vi "LV to ITX  Retrieve Equation.vi"(0 "File or Folder Path":path=path "\\\\TILES\\Data/SA02777G.graphene.20150414/12 - sweep B +-2T, step Vsg", 5 "offset":i32, 7 "length":i32=10, 9 "index":T1={"a"=3, "b"=5, "c"=7, "d"=9, "f"=2, "N1"=2, "N2"=0, "N3"=0, "N4"=0}) -> (4 "y1 vs f":cluster{dbl[], dbl[]}[](graph), 6 "y2 vs f":cluster{dbl[], dbl[]}[](graph), 8 "2D":dbl[][](graph), 10 "N":cluster{"N1":dbl, "N2":dbl, "N3":dbl, "N4":dbl}={"N1"=0.0, "N2"=3512286493.887331, "N3"=3512286493.887331, "N4"=3512286493.887331} {"N4" format="%#_6p"; "N3" format="%#_6p"; "N2" format="%#_6p"; "N1" format="%#_6p"}, 14 "Comments":string="sweep Vsg (22): 750mV to -500mV 50mV steps\r\n\r\n\r\n\r\n\r\n\r\n\r\n\r\n\r\n\r\n\r\n\r\n\r\n\r\n\r\nB=0T to 2T to -2T to 0T, 0.0104 A/s\r\n\r\n\r\n\r\n\r\n\r\n\r\n\r\n\r\n\r\n\r\n\r\n\r\n\r\n\r\n\r\n\r\n\r\n\r\n\r\n\r\n\r\n\r\n\r\n\r\n\r\n\r\n\r\n\r\n\r\nlockin\r\n\r\n\r\n\r\n\r\n\r\n\r\n\r\n\r\n\r\n\r\n\r\n\r\n\r\n\r\n0: 1\r\n\r\n\r\n\r\n\r\n\r\n\r\n\r\n\r\n\r\n\r\n\r\n\r\n\r\n\r\n1: 3\r\n\r\n\r\n\r\n\r\n\r\n\r\n\r\n\r\n\r\n\r\n\r\n\r\n\r\n\r\n2: 4, current\r\n\r\n\r\n\r\n\r\n\r\n\r\n\r\n\r\n\r\n\r\n\r\n\r\n\r\n\r\n3: 5\r\n\r\n\r\n\r\n\r\n\r\n\r\n\r\n\r\n\r\n\r\n\r\n\r\n\r\n\r\n4: 27\r\n\r\n\r\n\r\n\r\n\r\n\r\n\r\n\r\n\r\n\r\n\r\n\r\n\r\n\r\n5: 28, current, 8mV AC\r\n\r\n\r\n\r\n\r\n\r\n\r\n\r\n\r\n\r\n\r\n\r\n\r\n\r\n\r\nappliedVsg= 0.300000\r\n\r\n\r\n\r\n\r\n\r\n\r\n\r\n\r\n\r\n\r\n\r\n\r\n\r\n\r\n")   [LabVIEW 2013]
uses:
  <vilib>/Utility/miscctls.llb/LVOffsetAndMultiplierTypeDef.ctl
  <vilib>/gmath/NI_Gmath.lvlib
panel:
  in  "2D graph:\non = y1, off = y2":bool=TRUE
  in  "reverse arrays?":bool[](array[boolean])
  in  "header length":i32=11
  in  "Normalize MR?":bool=TRUE
  in  "threshold y":dbl
  in  "data length":i32=2500
  in  "data index":i32=1400
  in  "string formula = ON\nblock diagram formula = OFF":bool
  in  "Enum":enum16{"ITX", "ITX w/ 2D", "DAT"}(ring)=enum."DAT"
  in  "formula":string="y1 = (a-b)/c;\ny2 = (b-d)/c;"
  in  "D  is time?":bool
  in  "B is time?":bool
  out "time":string[][](table)=[["4/18/2015", "12:40 PM"], ["4/18/2015", "5:05 PM"], ["4/18/2015", "10:04 PM"], ["4/18/2015", "11:37 PM"], ["4/19/2015", "1:07 AM"], ["4/19/2015", "2:37 AM"], ["4/19/2015", "4:07 AM"], ["4/19/2015", "5:37 AM"], ["4/19/2015", "7:08 AM"], ["4/19/2015", "8:38 AM"]]
  in  "Use Folder Index File?":bool
  in  "Generate Folder Index File?":bool
  in  "Ez name":string="Ez name"
  in  "Ey name":string="Ey name"
  in  "Ex name":string="Ex name"
  in  "C y name":string="C y name"
  in  "D x name":string="D x name"
  in  "A y name":string="A y name"
  in  "B x name":string="B x name"
  out "Index, Wavenames":string[][](table)=[["0", "time"], ["1", "temp"], ["2", "Bfield"], ["3", "X0"], ["4", "Y0"], ["5", "X1"], ["6", "Y1"], ["7", "X2"], ["8", "Y2"], ["9", "X3"], ["10", "Y3"], ["11", "X4"], ["12", "Y4"], ["13", "X5"], ["", "Y5"]]
  in  "recolor traces?":bool=TRUE
  in  "Ex":T2={"Offset"=0.0, "Multiplier"=1.0}
  in  "Ey":T2={"Offset"=0.0, "Multiplier"=1.0}
  out "Path":path=path "\\\\TILES\\Data/SA02777G.graphene.20150414/12 - sweep B +-2T, step Vsg/SA02777G.graphene.20150414.000009.dat"
  out "counter":i32=9
  in  "pattern":string="*.dat"
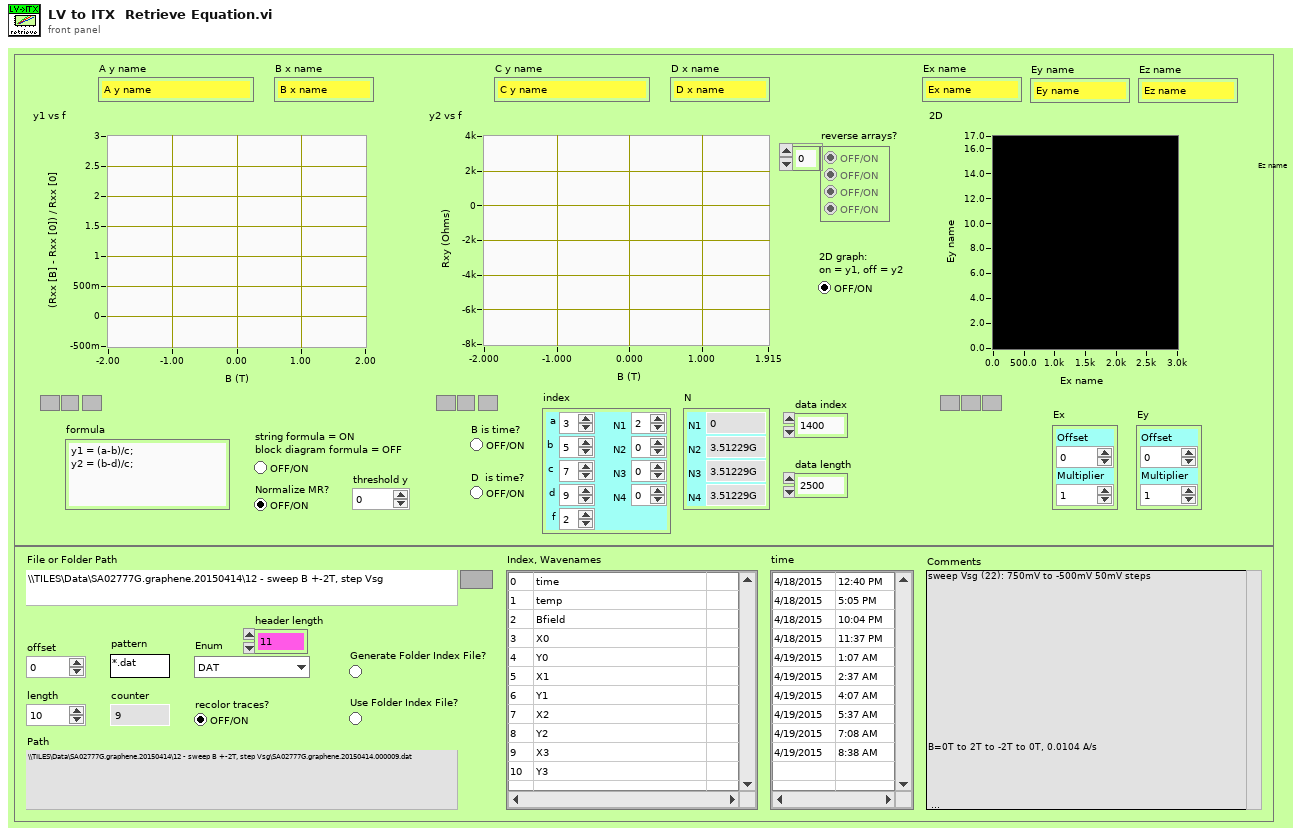
[diagram p1: front panel]
types:
  T1 = cluster{"a":i32, "b":i32, "c":i32, "d":i32, "f":i32, "N1":i32, "N2":i32, "N3":i32, "N4":i32}
  T2 = typedef "LVOffsetAndMultiplierTypeDef.ctl" = cluster{"Offset":dbl, "Multiplier":dbl}
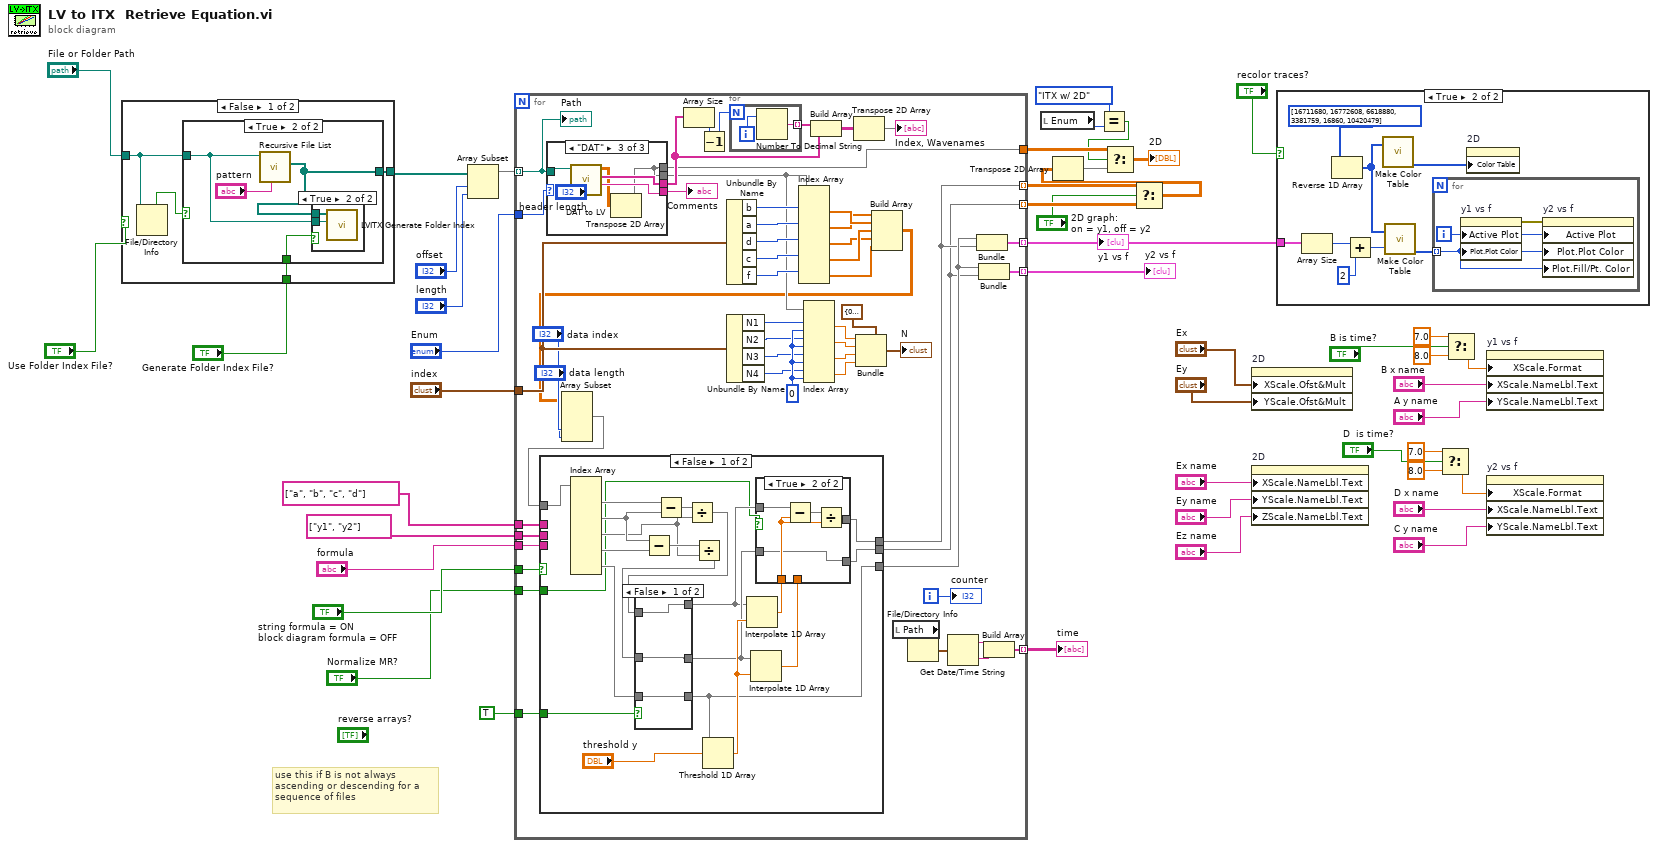
[diagram p0: block diagram]
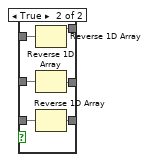
[diagram p3: hidden frame]
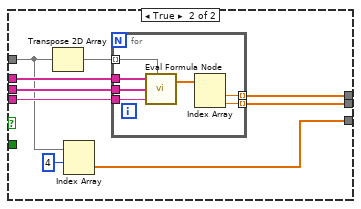
[diagram p5: hidden frame]
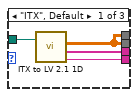
[diagram p6: hidden frame]
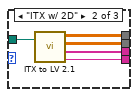
[diagram p7: hidden frame]
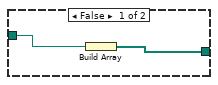
[diagram p8: hidden frame]
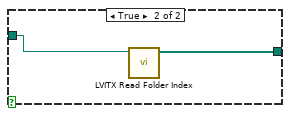
[diagram p10: hidden frame]
diagram:
  # "use this if B is not always\nascending or descending for a \nsequence of files"
  n1 = case shown="False" "Use Folder Index File?" {
    tunnel: [w48 w59] -> w44
    tunnel: "File or Folder Path" -> [w50 w60]
    tunnel: "Generate Folder Index File?" -> [w47 _]
    frame False {
      n2 = File/Directory Info(path=w50) -> (directory=w49:bool)  [unwired: 1 in, 6 out]
      n3 = case shown="True" w49 {
        tunnel: [w52 w55] -> w48
        tunnel: w50 -> [w51 w54]
        tunnel: w47 -> [_ w53]
        frame False {
          n4 = Build Array(w51) -> (w52:path[])
        }
        frame True {
          n5 = call <vilib>:"Recursive File List.vi"("pattern"="pattern", "Folder Path"=w54) -> ("All Files in Dir"=w55:path[])  [unwired: 5 in, 4 out]
          n6 = case shown="True" w53 {
            tunnel: w55 -> [_ w58]
            tunnel: w54 -> [_ w57]
            frame False {
            }
            frame True {
              n7 = call "LVITX Generate Folder Index.vi"("File or Folder Path"=w57, "All Files in Dir"=w58) -> ()  [unwired: 10 in]
            }
          }
        }
      }
    }
    frame True {
      n8 = call "LVITX Read Folder Index.vi"("File or Folder Path"=w60) -> ("Array"=w59:path[])  [unwired: 10 in]
    }
  }
  n9 = Array Subset(array=w44, index="offset", length="length") -> (w24:path[])
  n10 = for {
    tunnel: w24 -> [w112] mode=indexing
    tunnel: [w112] -> _ mode=indexing
    tunnel: [w111] -> w12 mode=indexing
    tunnel: [w110] -> w35 mode=indexing
    tunnel: [w103] -> w37
    tunnel: [w88] -> w27 mode=indexing
    tunnel: "formula" -> [w77]
    tunnel: string[] ["y1", "y2"] ("Variables Output") -> [w76]
    tunnel: string[] ["a", "b", "c", "d"] ("Variables Input") -> [w75]
    tunnel: "Enum" -> [w74]
    tunnel: "index" -> [w73]
    tunnel: "string formula = ON\nblock diagram formula = OFF" -> [w72]
    tunnel: "Normalize MR?" -> [w64]
    tunnel: TRUE ("Normalize MR? 2") -> [w63]
    tunnel: [w62] -> w4 mode=indexing
    tunnel: [w61] -> w2 mode=indexing
    i -> [w114]
    w102 = 0 ("disabled index (col)")
    n11 = case shown="\"DAT\"" w74 {
      tunnel: [w173 w176 w183] -> w113
      tunnel: [w171 w177 w180] -> w78
      tunnel: w112 -> [w172 w178 w184]
      tunnel: [w170 w175 w182] -> w104
      tunnel: [w171 w174 w180] -> w103
      frame "ITX", Default {
        n12 = call "ITX to LV 2.1 1D.vi"("file (use dialog)"=w172) -> ("1D arrays"=w171:dbl[][], "wave names"=w170:string[], "Notes"=w173:string)  [unwired: 2 in]
      }
      frame "ITX w/ 2D" {
        n13 = call "ITX to LV 2.1.vi"("file (use dialog)"=w178) -> ("2D array"=w174:dbl[][], "1D arrays"=w177:dbl[][], "wave names"=w175:string[], "Notes"=w176:string)  [unwired: 1 in]
      }
      frame "DAT" {
        n14 = call "DAT to LV.vi"("header length"="header length", "File Path"=w184) -> ("Comments"=w183:string, "Wavenames"=w182:string[], "Data"=w181:dbl[][])  [unwired: 7 in]
        n15 = Transpose 2D Array(2D array=w181) -> (transposed array=w180:dbl[][])
      }
    }
    "Comments" <- w113
    n16 = Array Size(array=w104) -> (size(s)=w107:i32)
    n17 = Decrement(x=w107) -> (x-1=w106:i32)
    n18 = Unbundle By Name(w73) -> ("b"=w96:i32, "a"=w95:i32, "d"=w94:i32, "c"=w93:i32, "f"=w80:i32)
    n19 = Unbundle By Name(w73) -> ("N1"=w97:i32, "N2"=w98:i32, "N3"=w99:i32, "N4"=w100:i32)
    n20 = for {
      N: w106 -> [_]
      tunnel: [w168] -> w109 mode=indexing
      i -> [w169]
      n21 = Number To Decimal String(number=w169) -> (decimal integer string=w168:string)  [unwired: 1 in]
    }
    n22 = Index Array(array=w78, index (row) #1=w96, index (row) #2=w95, index (row) #3=w94, index (row) #4=w93, index (row) #5=w80) -> (element #1=w87:dbl[], element #2=w81:dbl[], element #3=w79:dbl[], element #4=w86:dbl[], element #5=w68:dbl[])  [unwired: 5 in]
    n23 = Index Array(array=w78, index (row) #1=w97, index (col) #1=w102, index (row) #2=w98, index (col) #2=w102, index (row) #3=w99, index (col) #3=w102, index (row) #4=w100, index (col) #4=w102) -> (element #1=w85:dbl, element #2=w84:dbl, element #3=w83:dbl, element #4=w82:dbl)
    n24 = Build Array(w109, w104) -> (w105:string[][])
    n25 = Transpose 2D Array(2D array=w105) -> (transposed array=→"Index, Wavenames":string[][])
    n26 = Bundle(cluster=cluster{"N1":dbl, "N2":dbl, "N3":dbl, "N4":dbl} {"N1"=0.0, "N2"=0.0, "N3"=0.0, "N4"=0.0}, "N1"=w85, "N2"=w84, "N3"=w83, "N4"=w82) -> (→"N":cluster{"N1":dbl, "N2":dbl, "N3":dbl, "N4":dbl})
    n27 = Build Array(w81, w87, w86, w79, w68) -> (w67:dbl[][])
    n28 = Array Subset(array=w67, index (col)="data index", length (col)="data length") -> (w66:dbl[][])  [unwired: 2 in]
    n29 = case shown="False" w72 {
      tunnel: [w118 w160] -> w61
      tunnel: w66 -> [w135 w154]
      tunnel: [w117 w159] -> w62
      tunnel: w77 -> [_ w158]
      tunnel: w76 -> [_ w157]
      tunnel: w75 -> [_ w156]
      tunnel: [w124 w152] -> w65
      tunnel: w64 -> [w116 _]
      tunnel: w63 -> [w115 _]
      frame False {
        n30 = Index Array(array=w135) -> (element #1=w134:dbl[], element #2=w133:dbl[], element #3=w129:dbl[], element #4=w132:dbl[], element #5=w127:dbl[])  [unwired: 10 in]
        n31 = Subtract(x=w133, y=w132) -> (x-y=w130:dbl[])
        n32 = Subtract(x=w134, y=w133) -> (x-y=w131:dbl[])
        n33 = Divide(x=w131, y=w129) -> (x/y=w128:dbl[])
        n34 = Divide(x=w130, y=w129) -> (x/y=w123:dbl[])
        n35 = case shown="False" w115 {
          tunnel: w128 -> [w138 w144]
          tunnel: w127 -> [w136 w143]
          tunnel: [w136 w142] -> w124
          tunnel: w123 -> [w137 w141]
          tunnel: [w137 w140] -> w120
          tunnel: [w138 w139] -> w119
          frame False {
          }
          frame True {
            n36 = Reverse 1D Array(array=w144) -> (reversed array=w139:dbl[])
            n37 = Reverse 1D Array(array=w141) -> (reversed array=w140:dbl[])
            n38 = Reverse 1D Array(array=w143) -> (reversed array=w142:dbl[])
          }
        }
        n39 = Threshold 1D Array(2:"threshold y", 3:w124) -> (0:w125:dbl)  [unwired: 1 in]
        n40 = Interpolate 1D Array(1:w125, 2:w119) -> (0:w121:dbl)
        n41 = Interpolate 1D Array(1:w125, 2:w120) -> (0:w122:dbl)
        n42 = case shown="True" w116 {
          tunnel: w122 -> [_ _]
          tunnel: w121 -> [_ w151]
          tunnel: w120 -> [w145 w147]
          tunnel: w119 -> [w146 w150]
          tunnel: [w145 w147] -> w118
          tunnel: [w146 w148] -> w117
          frame False {
          }
          frame True {
            n43 = Subtract(x=w150, y=w151) -> (x-y=w149:dbl[])
            n44 = Divide(x=w149, y=w151) -> (x/y=w148:dbl[])
          }
        }
      }
      frame True {
        n45 = Transpose 2D Array(2D array=w154) -> (transposed array=w155:dbl[][])
        n46 = Index Array(array=w154, index (row)=4) -> (element=w152:dbl[])  [unwired: 1 in]
        n47 = for {
          tunnel: w156 -> [w167]
          tunnel: w157 -> [w166]
          tunnel: w158 -> [w165]
          tunnel: w155 -> [w161] mode=indexing
          tunnel: [w163] -> w160 mode=indexing
          tunnel: [w162] -> w159 mode=indexing
          n48 = call <vilib>:"Eval Formula Node.vi"("Variables Input"=w167, "Input Values"=w161, "Variables Output"=w166, "formula"=w165) -> ("Output Values"=w164:dbl[])  [unwired: 1 in, 1 out]
          n49 = Index Array(array=w164) -> (element #1=w162:dbl, element #2=w163:dbl)  [unwired: 2 in]
        }
      }
    }
    n50 = local read "Path"() -> (w92:path)
    n51 = File/Directory Info(path=w92) -> (last mod=w91:timestamp)  [unwired: 1 in, 6 out]
    n52 = Get Date/Time String(seconds (now)=w91) -> (date string=w90:string, time string=w89:string)  [unwired: 2 in]
    n53 = Bundle(w65, w62) -> (w111:cluster{dbl[], dbl[]})  [unwired: 1 in]
    n54 = Bundle(w65, w61) -> (w110:cluster{dbl[], dbl[]})  [unwired: 1 in]
    n55 = Build Array(w90, w89) -> (w88:string[])
    "counter" <- w114
    "Path" <- w112
  }
  "y1 vs f" <- w12
  "y2 vs f" <- w35
  "time" <- w27
  n56 = local read "Enum"() -> (w14:enum16{"ITX", "ITX w/ 2D", "DAT"})
  n57 = Equal?(x=enum16{"ITX", "ITX w/ 2D", "DAT"}."ITX w/ 2D" ("Enum"), y=w14) -> (x = y?=w13:bool)
  n58 = Select(t=w4, s="2D graph:\non = y1, off = y2", f=w2) -> (s? t:f=w3:dbl[][])
  n59 = Transpose 2D Array(2D array=w3) -> (transposed array=w39:dbl[][])
  n60 = Select(t=w37, s=w13, f=w39) -> (s? t:f=→"2D":dbl[][])
  n61 = property on="2D" class="IntGraph (strict)"("XScale.Ofst&Mult"="Ex", "YScale.Ofst&Mult"="Ey") -> ()  [unwired: 2 in, 2 out]
  n62 = property on="2D" class="IntGraph (strict)"("XScale.NameLbl.Text"="Ex name", "YScale.NameLbl.Text"="Ey name", "ZScale.NameLbl.Text"="Ez name") -> ()  [unwired: 2 in, 2 out]
  n63 = case shown="True" "recolor traces?" {
    tunnel: w12 -> [_ w187]
    frame False {
    }
    frame True {
      n64 = Array Size(array=w187) -> (size(s)=w188:i32)
      n65 = Reverse 1D Array(array=u32[] [16711680, 16772608, 6618880, 3381759, 16860, 10420479] ("color scale")) -> (reversed array=w186:u32[])
      n66 = Add(x=w188, y=2 ("x")) -> (x+y=w192:i32)
      n67 = call <userlib>:"Make Color Table.vi"("Array"=w186) -> ("Color Tbl"=w190:u32[])  [unwired: 1 in, 3 out]
      n68 = call <userlib>:"Make Color Table.vi"("Array"=w186, "Size/3"=w192) -> ("Color Tbl"=w189:u32[])  [unwired: 3 out]
      n69 = for {
        tunnel: w189 -> [w193] mode=indexing
        i -> [w194]
        n70 = property on="y1 vs f" class="XYGraph (strict)"("Active Plot"=w194, "Plot.Plot Color"=w193) -> (error out=w195:errorcluster)  [unwired: 2 in, 1 out]
        n71 = property on="y2 vs f" class="XYGraph (strict)"(error in=w195, "Active Plot"=w194, "Plot.Plot Color"=w193, "Plot.Fill/Pt. Color"=w193) -> ()  [unwired: 1 in, 2 out]
      }
      n72 = property on="2D" class="IntGraph (strict)"("Color Table"=w190) -> ()  [unwired: 2 in, 2 out]
    }
  }
  n73 = Select(t=7.0, s="D  is time?", f=8.0) -> (s? t:f=w20:dbl)
  n74 = Select(t=7.0, s="B is time?", f=8.0) -> (s? t:f=w21:dbl)
  n75 = property on="y1 vs f" class="XYGraph (strict)"("XScale.Format"=w21, "XScale.NameLbl.Text"="B x name", "YScale.NameLbl.Text"="A y name") -> ()  [unwired: 2 in, 2 out]
  n76 = property on="y2 vs f" class="XYGraph (strict)"("XScale.Format"=w20, "XScale.NameLbl.Text"="D x name", "YScale.NameLbl.Text"="C y name") -> ()  [unwired: 2 in, 2 out]
